vi "表格清空.vi"(9 "数值":i32, 10 "电压输出电流传感器测试":refnum<vi>, 11 "电流传感器测试":refnum<vi>) -> (2 "电压输出电流传感器测试 2":refnum<vi>, 3 "电流传感器测试 2":refnum<vi>)   [LabVIEW 2021]
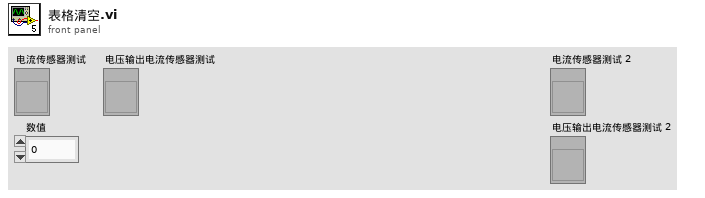
[diagram p1: front panel]
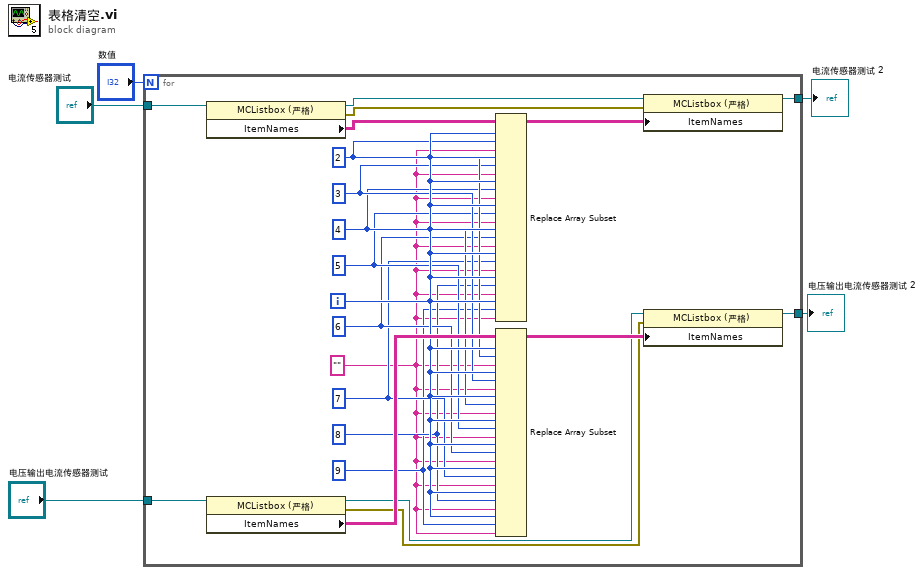
[diagram p0: block diagram]
diagram:
  n1 = for {
    N: "数值" -> [_]
    tunnel: "电流传感器测试" -> [w17]
    tunnel: [w16] -> w3
    tunnel: "电压输出电流传感器测试" -> [w19]
    tunnel: [w18] -> w2
    i -> [w15]
    w6 = "" ("新元素/子数组")
    w7 = 9
    w8 = 8
    w9 = 7
    w10 = 6
    w11 = 5
    w12 = 4
    w13 = 3
    w14 = 2
    n2 = property class="MCListbox (严格)"(reference=w17) -> (reference out=w26:refnum<vi>, error out=w24:errorcluster, "ItemNames"=w27:string[][])  [unwired: 1 in]
    n3 = property class="MCListbox (严格)"(reference=w19) -> (reference out=w21:refnum<vi>, error out=w20:errorcluster, "ItemNames"=w23:string[][])  [unwired: 1 in]
    n4 = Replace Array Subset(array=w27, new element #1=w6, index (row) #1=w15, index (col) #1=w14, new element #2=w6, index (row) #2=w15, index (col) #2=w13, new element #3=w6, index (row) #3=w15, index (col) #3=w12, new element #4=w6, index (row) #4=w15, index (col) #4=w11, new element #5=w6, index (row) #5=w15, index (col) #5=w10, new element #6=w6, index (row) #6=w15, index (col) #6=w9, new element #7=w6, index (row) #7=w15, index (col) #7=w8, new element #8=w6, index (row) #8=w15, index (col) #8=w7) -> (w25:string[][])
    n5 = Replace Array Subset(array=w23, new element #1=w6, index (row) #1=w15, index (col) #1=w14, new element #2=w6, index (row) #2=w15, index (col) #2=w13, new element #3=w6, index (row) #3=w15, index (col) #3=w12, new element #4=w6, index (row) #4=w15, index (col) #4=w11, new element #5=w6, index (row) #5=w15, index (col) #5=w10, new element #6=w6, index (row) #6=w15, index (col) #6=w9, new element #7=w6, index (row) #7=w15, index (col) #7=w8, new element #8=w6, index (row) #8=w15, index (col) #8=w7) -> (w22:string[][])
    n6 = property class="MCListbox (严格)"(reference=w26, error in=w24, "ItemNames"=w25) -> (reference out=w16:refnum<vi>)  [unwired: 1 out]
    n7 = property class="MCListbox (严格)"(reference=w21, error in=w20, "ItemNames"=w22) -> (reference out=w18:refnum<vi>)  [unwired: 1 out]
  }
  "电流传感器测试 2" <- w3
  "电压输出电流传感器测试 2" <- w2
